vi "create discrete histogram.vi"(1 "Array in":i16[](array[numeric])) -> (0 "Array out":cluster{i32[], i16[]}(graph))   [LabVIEW 2009]
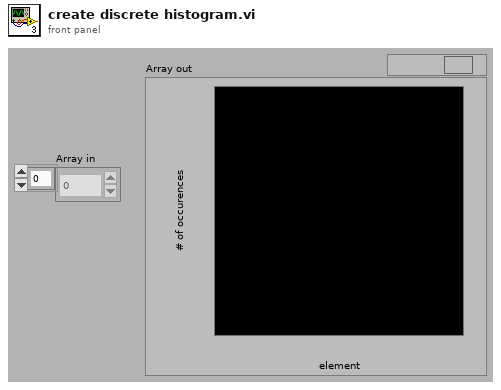
[diagram p1: front panel]
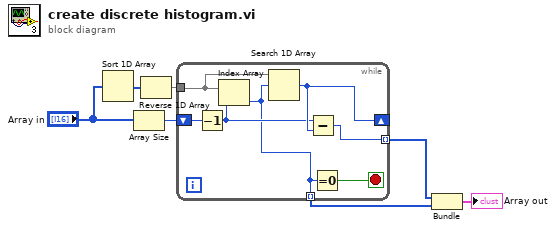
[diagram p0: block diagram]
diagram:
  n1 = Sort 1D Array(array="Array in") -> (sorted array=w4:i16[])
  n2 = Array Size(array="Array in") -> (size(s)=w6:i32)
  n3 = Reverse 1D Array(array=w4) -> (reversed array=w5:i16[])
  n4 = while {
    tunnel: w5 -> [w14]
    shift-right: [w12] -> _
    shift-left: w6 -> [w13]
    tunnel: [w9] -> w2 mode=indexing
    tunnel: [w8] -> w3 mode=indexing
    stop <- w10 stop-if-true
    n5 = Decrement(x=w13) -> (x-1=w11:i32)
    n6 = Index Array(array=w14, index=w11) -> (element=w9:i16)
    n7 = Search 1D Array(1D array=w14, element=w9) -> (index of element=w12:i32)  [unwired: 1 in]
    n8 = Subtract(x=w11, y=w12) -> (x-y=w8:i32)
    n9 = Equal To 0?(x=w9) -> (x = 0?=w10:bool)
  }
  n10 = Bundle(w3, w2) -> (→"Array out":cluster{i32[], i16[]})  [unwired: 1 in]
